vi "SetStatisticalData.vi"(8 "error in (no error)":errorcluster caption="错误输入（无错误）", 10 "组合框":string(combo), 11 "configuration file path":path caption="配置文件的路径") -> (0 "error out":errorcluster caption="错误输出", 2 "value":string, 3 "configuration file path 2":path)   [LabVIEW 2018]
uses:
  <vilib>/Utility/config.llb/Read Key (String).vi
  <vilib>/Utility/config.llb/Write Key (String).vi
  <vilib>/Utility/config.llb/NI_LVConfig.lvlib
panel:
  out "key names":string[](array[string]) caption="键名"
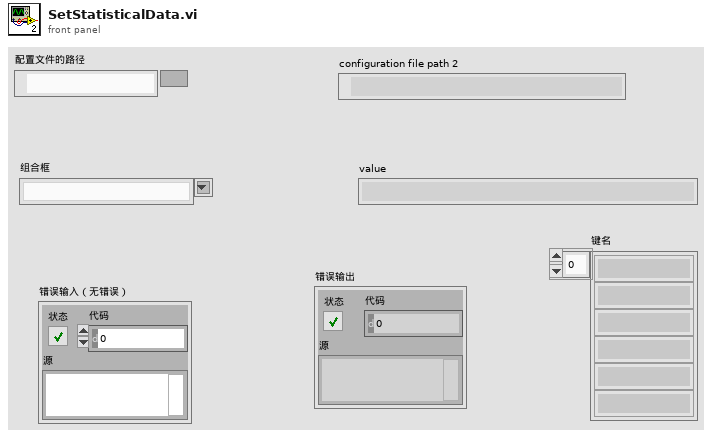
[diagram p1: front panel]
types:
  T1 = typedef "NI_LVConfig.lvlib/Config Data RefNum.ctl" = refnum<k1>
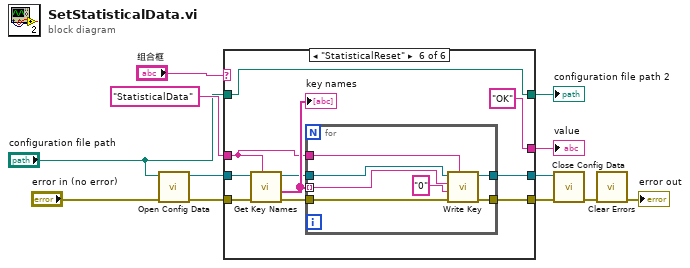
[diagram p0: block diagram]
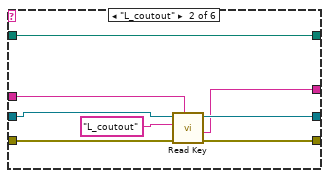
[diagram p3: hidden frame]
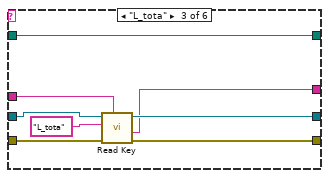
[diagram p4: hidden frame]
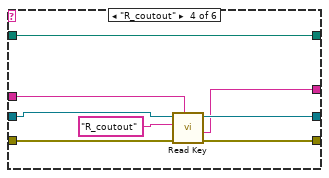
[diagram p5: hidden frame]
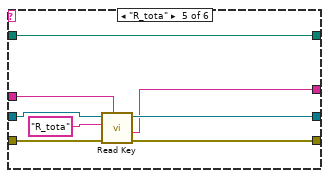
[diagram p6: hidden frame]
diagram:
  n1 = call <vilib>:"Open Config Data.vi"("error in (no error)"="error in (no error)", "configuration file path"="configuration file path") -> ("error out"=w3:errorcluster, "refnum"=w11:T1)  [unwired: 7 in, 1 out]
  n2 = case shown="\"StatisticalReset\"" "组合框" {
    tunnel: w11 -> [w14 w23 w31 w39 w47 w57]
    tunnel: "StatisticalData" -> [_ w22 w30 w38 w46 w48]
    tunnel: [w14 w20 w28 w36 w44 w50] -> w9
    tunnel: [_ w19 w27 w35 w43 "OK" ("value")] -> w8
    tunnel: [w15 w18 w26 w34 w42 w55] -> w6
    tunnel: "configuration file path" -> [w15 w18 w26 w34 w42 w55]
    tunnel: [w13 w17 w24 w33 w40 w51] -> w4
    tunnel: w3 -> [w13 w16 w25 w32 w41 w56]
    frame "假", Default {
    }
    frame "L_coutout" {
      n3 = call-poly <vilib>:"Read Key.vi"("section"=w22, "error in (no error)"=w16, "key"="L_coutout", "refnum"=w23) -> ("error out"=w17:errorcluster, "value"=w19:string, "refnum out"=w20:T1)  [unwired: 4 in, 1 out]
    }
    frame "L_tota" {
      n4 = call-poly <vilib>:"Read Key.vi"("section"=w30, "error in (no error)"=w25, "key"="L_tota", "refnum"=w31) -> ("error out"=w24:errorcluster, "value"=w27:string, "refnum out"=w28:T1)  [unwired: 4 in, 1 out]
    }
    frame "R_coutout" {
      n5 = call-poly <vilib>:"Read Key.vi"("section"=w38, "error in (no error)"=w32, "key"="R_coutout", "refnum"=w39) -> ("error out"=w33:errorcluster, "value"=w35:string, "refnum out"=w36:T1)  [unwired: 4 in, 1 out]
    }
    frame "R_tota" {
      n6 = call-poly <vilib>:"Read Key.vi"("section"=w46, "error in (no error)"=w41, "key"="R_tota", "refnum"=w47) -> ("error out"=w40:errorcluster, "value"=w43:string, "refnum out"=w44:T1)  [unwired: 4 in, 1 out]
    }
    frame "StatisticalReset" {
      n7 = call <vilib>:"Get Key Names.vi"("section"=w48, "error in (no error)"=w56, "refnum"=w57) -> ("error out"=w54:errorcluster, "key names"=w53:string[], "refnum out"=w52:T1)  [unwired: 5 in, 1 out]
      "key names" <- w53
      n8 = for {
        tunnel: w54 -> [w64]
        tunnel: w53 -> [w63] mode=indexing
        tunnel: w52 -> [w62]
        tunnel: [w60] -> w51
        tunnel: [w59] -> w50
        tunnel: w48 -> [w58]
        n9 = call-poly <vilib>:"Write Key.vi"("section"=w58, "error in (no error)"=w64, "value"="0", "key"=w63, "refnum"=w62) -> ("error out"=w60:errorcluster, "refnum out"=w59:T1)  [unwired: 4 in, 1 out]
      }
    }
  }
  "value" <- w8
  "configuration file path 2" <- w6
  n10 = call <vilib>:"Close Config Data.vi"("error in (no error)"=w4, "refnum"=w9) -> ("error out"=w5:errorcluster)  [unwired: 8 in, 1 out]
  n11 = call <vilib>:"Clear Errors.vi"("error in (no error)"=w5) -> ("error out"=→"error out":errorcluster)  [unwired: 5 in, 1 out]
